vi "donut Animate.vi"() -> ()   [LabVIEW 2011]
doc: "This VI demonstrates how to animate a picture on the front panel using a picture ring (Pict Ring) control. This VI takes a sequence of pictures where each picture represents a \"frame\" of the animaction and makes each picture a selection in the picture ring. By programmatically incrementing the value of the picture ring, the picture appears to be animated."
panel:
  in  "停止":bool
  in  "等待时间（毫秒）":u32=100
  out "donut":picture
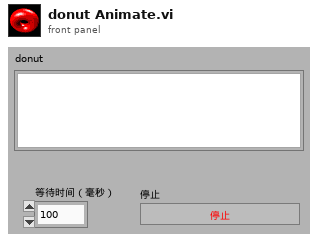
[diagram p1: front panel]
types:
  T1 = typedef "LVBoundsTypeDef.ctl" = cluster{"Width":u32, "Height":u32}
  T2 = cluster{"left":i16, "top":i16, "right":i16, "bottom":i16}
  T3 = typedef "imagedata.ctl" = cluster{"image type":i32, "image depth":i32, "image":u8[], "mask":u8[], "colors":u32[], "Rectangle":cluster{"left":i16, "top":i16, "right":i16, "bottom":i16}}
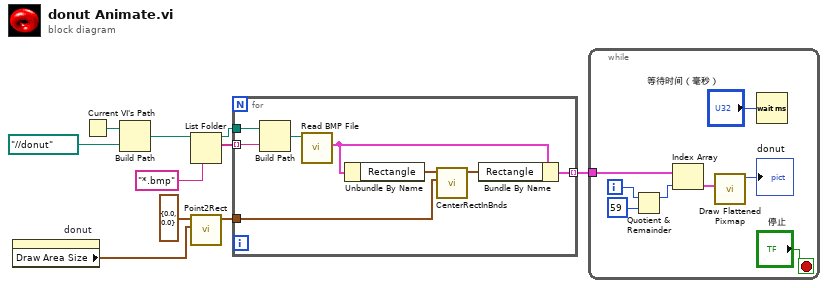
[diagram p0: block diagram]
diagram:
  n1 = property on="donut" class="Pict"() -> ("Draw Area Size"=w10:T1)  [unwired: 2 in, 2 out]
  n2 = Current VI's Path() -> (path=w8:path)
  n3 = Build Path(base path=w8, name or relative path=path "../../donut" ("基路径")) -> (appended path=w4:path)
  n4 = List Folder(path=w4, pattern="*.bmp" ("模式")) -> (path out=w1:path, filenames=w5:string[])  [unwired: 2 in, 2 out]
  n5 = call "Point2Rect.vi"("point b"=w10, "point a"=cluster{"x":dbl, "y":dbl} {"x"=0.0, "y"=0.0}) -> ("rect"=w2:T2)  [unwired: 8 in, 1 out]
  n6 = for {
    tunnel: w5 -> [w17] mode=indexing
    tunnel: w1 -> [w18]
    tunnel: [w13] -> w3 mode=indexing
    tunnel: w2 -> [w16]
    n7 = Build Path(base path=w18, name or relative path=w17) -> (appended path=w11:path)
    n8 = call <vilib>:"Read BMP File.vi"("path to BMP file"=w11) -> ("image data"=w15:T3)  [unwired: 8 in, 2 out]
    n9 = Unbundle By Name(w15) -> ("Rectangle"=w14:T2)
    n10 = call "CenterRectInBnds.vi"("bounds"=w16, "rect"=w14) -> ("centered rect"=w12:T2)  [unwired: 8 in, 1 out]
    n11 = Bundle By Name(cluster=w15, "Rectangle"=w12) -> (w13:T3)
  }
  n12 = while {
    tunnel: w3 -> [w24]
    i -> [w26]
    stop <- "停止" stop-if-true
    n13 = Quotient & Remainder(x=w26, y=59) -> (x-y*floor(x/y)=w23:i32)  [unwired: 1 out]
    n14 = Index Array(array=w24, index=w23) -> (element=w22:T3)
    n15 = call <vilib>:"Draw Flattened Pixmap.vi"("image data"=w22) -> ("new picture"=→"donut":picture)  [unwired: 8 in]
    n16 = Wait (ms)(milliseconds to wait="等待时间（毫秒）") -> ()  [unwired: 1 out]
  }
